vi "Get SMO Public API.vi"(8 "error in (no error)":errorcluster, 11 "Instrument in":refnum<class "Instrument.lvclass">) -> (0 "error out":errorcluster, 2 "commands":string[](array[string]), 3 "Instrument out":refnum<class "Instrument.lvclass">)   [LabVIEW 2019, in "Instrument.lvclass"]
doc: "Override this VI to return a list of commands supported by your Instrument"
uses:
  Instrument.lvclass
  Instrument.lvclass/Instrument.ctl
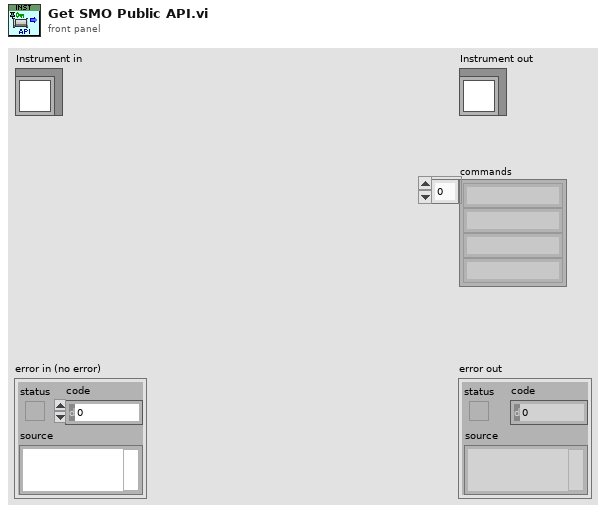
[diagram p1: front panel]
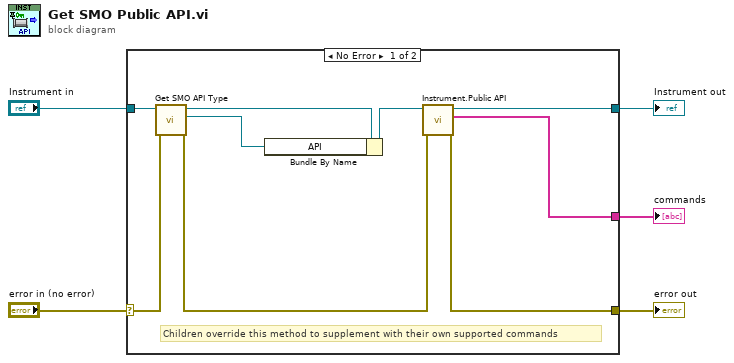
[diagram p0: block diagram]
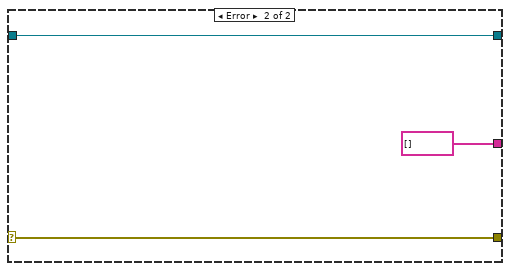
[diagram p2: hidden frame]
diagram:
  n1 = case shown="No Error" "error in (no error)" {
    selector: "error in (no error)" -> [w11 w17]
    tunnel: [w6 w17] -> w4
    tunnel: [w8 w16] -> w2
    tunnel: "Instrument in" -> [w13 w16]
    tunnel: [w10 string[] [] ("Array")] -> w1
    frame No Error {
      # "Children override this method to supplement with their own supported commands"
      n2 = call-dynamic "Get SMO API Type.vi"("error in (no error)"=w11, "Instrument in"=w13) -> ("error out"=w7:errorcluster, "API"=w12:refnum<class "API.lvclass">, "Instrument out"=w14:refnum<class "Instrument.lvclass">)  [unwired: 7 in]
      n3 = Bundle By Name(cluster=w14, "API"=w12) -> (w9:refnum<class "Instrument.lvclass">)
      n4 = call "Instrument.Public API.vi"("error in (no error)"=w7, "Instrument in"=w9) -> ("error out"=w6:errorcluster, "commands (this level)"=w10:string[], "Instrument out"=w8:refnum<class "Instrument.lvclass">)  [unwired: 7 in]
    }
    frame Error {
    }
  }
  "error out" <- w4
  "Instrument out" <- w2
  "commands" <- w1
